vi "Main.vi"() -> ()   [LabVIEW 2019]
uses:
  <vilib>/addons/zeromq/socket_type.ctl
  <vilib>/FPGAPlugInAG/myRIO-1900/niLvFpga_Open_myRIO-1900.vi
  <vilib>/rvi/interface/common/dynamic/niFpgaDynamicAddResources.vi
  <vilib>/Utility/error.llb/Error Cluster From Error Code.vi
  <vilib>/rvi/errors/niLvFpgaAdjustHostInterfaceError.vi
  <vilib>/rvi/interface/nirviOpenFPGA/nirviOpenFPGA.xnode
  FPGA Bitfiles/hybridpulser_FPGATarget_fpgamainfsm_024CIbEM8OY.lvbitx
  <vilib>/rvi/interface/nirviMethod/nirviMethod.xnode
  <vilib>/FPGAPlugInAG/Dynamic/niLvFpga_WriteFifo_Dynamic.vi
  <vilib>/rvi/errors/niLvFpgaMergeErrorWithErrorCode.vi
  <vilib>/addons/zeromq/zmq_context.lvclass
  <vilib>/addons/zeromq/zeromq.lvlib
  <vilib>/addons/zeromq/zmq_socket.lvclass
panel:
  out "progs":i32
  out "output array":u32[](array[numeric])
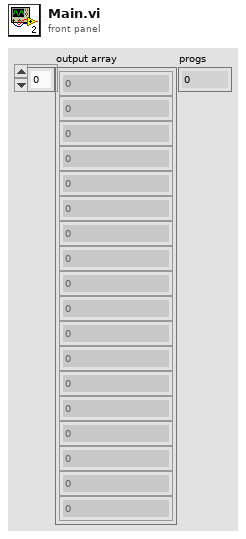
[diagram p1: front panel]
types:
  T1 = typedef "zeromq.lvlib/socket_type.ctl" = enum8{"ZMQ_PAIR", "ZMQ_PUB", "ZMQ_SUB", "ZMQ_REQ", "ZMQ_REP", "ZMQ_DEALER", "ZMQ_ROUTER", "ZMQ_PULL", "ZMQ_PUSH", "ZMQ_XPUB", "ZMQ_XSUB"}
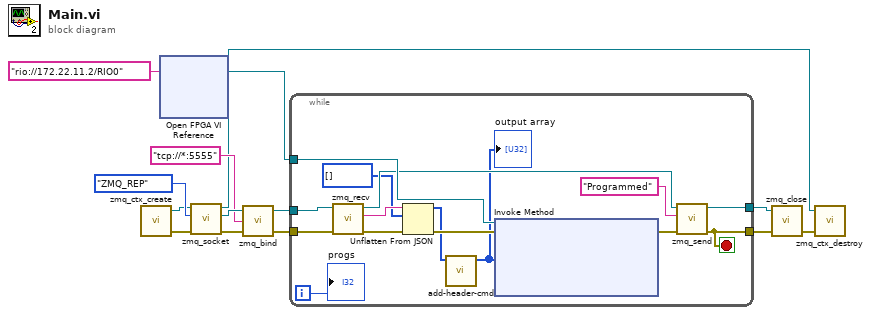
[diagram p0: block diagram]
diagram:
  n1 = call <vilib>:"zmq_ctx_create.vi"() -> ("error out"=w12:errorcluster, "context out"=w13:refnum<class "zmq_context.lvclass">)  [unwired: 4 in]
  n2 = xnode "Open FPGA VI Reference"("resource name"=tag "rio://172.22.11.2/RIO0") -> ("FPGA VI Reference Out"=w6:refnum<k20>)  [unwired: 1 in, 1 out]
  n3 = call <vilib>:"zmq_socket.vi"("error in"=w12, "socket type"=socket_type."ZMQ_REP", "context in"=w13) -> ("error out"=w11:errorcluster, "socket out"=w10:refnum<class "zmq_socket.lvclass">, "context out"=w2:refnum<class "zmq_context.lvclass">)  [unwired: 2 in]
  n4 = call <vilib>:"zmq_bind.vi"("error in"=w11, "endpoint"="tcp://*:5555", "socket in"=w10) -> ("error out"=w7:errorcluster, "socket out"=w8:refnum<class "zmq_socket.lvclass">)  [unwired: 1 in]
  n5 = while {
    tunnel: w8 -> [w29]
    tunnel: w7 -> [w28]
    tunnel: w6 -> [w26]
    tunnel: [w20] -> w5
    tunnel: [w19] -> w4
    i -> [w15]
    stop <- w19 stop-if-true
    n6 = call <vilib>:"zmq_recv.vi"("error in"=w28, "socket in"=w29) -> ("error out"=w25:errorcluster, "data"=w27:string, "socket out"=w21:refnum<class "zmq_socket.lvclass">)  [unwired: 3 in, 2 out]
    n7 = Unflatten From JSON(JSON string=w27, type and defaults=u32[] [] ("Data"), error in (no error)=w25) -> (value=w17:u32[], error out=w24:errorcluster)  [unwired: 4 in]
    n8 = call "add-header-cmd"("Data in"=w17) -> ("Data out"=w16:u32[])  [unwired: 10 in]
    "output array" <- w16
    n9 = xnode "Invoke Method"("FPGA VI Reference In"=w26, "error in"=w24, "Data"=w16) -> ("error out"=w23:errorcluster)  [unwired: 1 in, 2 out]
    n10 = call <vilib>:"zmq_send.vi"("error in"=w23, "data"="Programmed", "socket in"=w21) -> ("error out"=w19:errorcluster, "socket out"=w20:refnum<class "zmq_socket.lvclass">)  [unwired: 4 in]
    "progs" <- w15
  }
  n11 = call <vilib>:"zmq_close.vi"("error in"=w4, "socket"=w5) -> ("error out"=w3:errorcluster)  [unwired: 3 in]
  n12 = call <vilib>:"zmq_ctx_destroy.vi"("error in"=w3, "context in"=w2) -> ()  [unwired: 3 in, 1 out]
